vi "Lambda_Configuration_ex_versao1.vi"() -> ()   [LabVIEW 2015]
uses:
  <vilib>/Utility/error.llb/DialogType.ctl
  <vilib>/Utility/file.llb/Read From Spreadsheet File (DBL).vi
  <vilib>/Utility/NIReport.llb/NI_report.lvclass
  <vilib>/addons/_office/NI_ReportGenerationToolkit.lvlib
panel:
  in  "LED Measurement":dbl
  out "error out":errorcluster
  in  "report file path":path=path "C:/Users/Tulio/Documents/Testes/Backup excel/backup excel.xlsx"
  out "Voltage":dbl[](graph)
  out "Current":dbl[](graph)
  in  "Load File?":bool
  in  "?":bool
  out "Output Current":dbl format="%.6f"
  out "Output Voltage":dbl format="%.6f"
  out "Serial Number:":string
  out "error?":bool
  out "Model:":string
  in  "Reset (T)":bool=TRUE
  in  "BAUD":u16(ring)=3 items=["1200", "2400", "4800", "9600", "19200"]
  in  "GEN Addr":i16=6
  in  "VISA name":refnum<visa-resource-name>
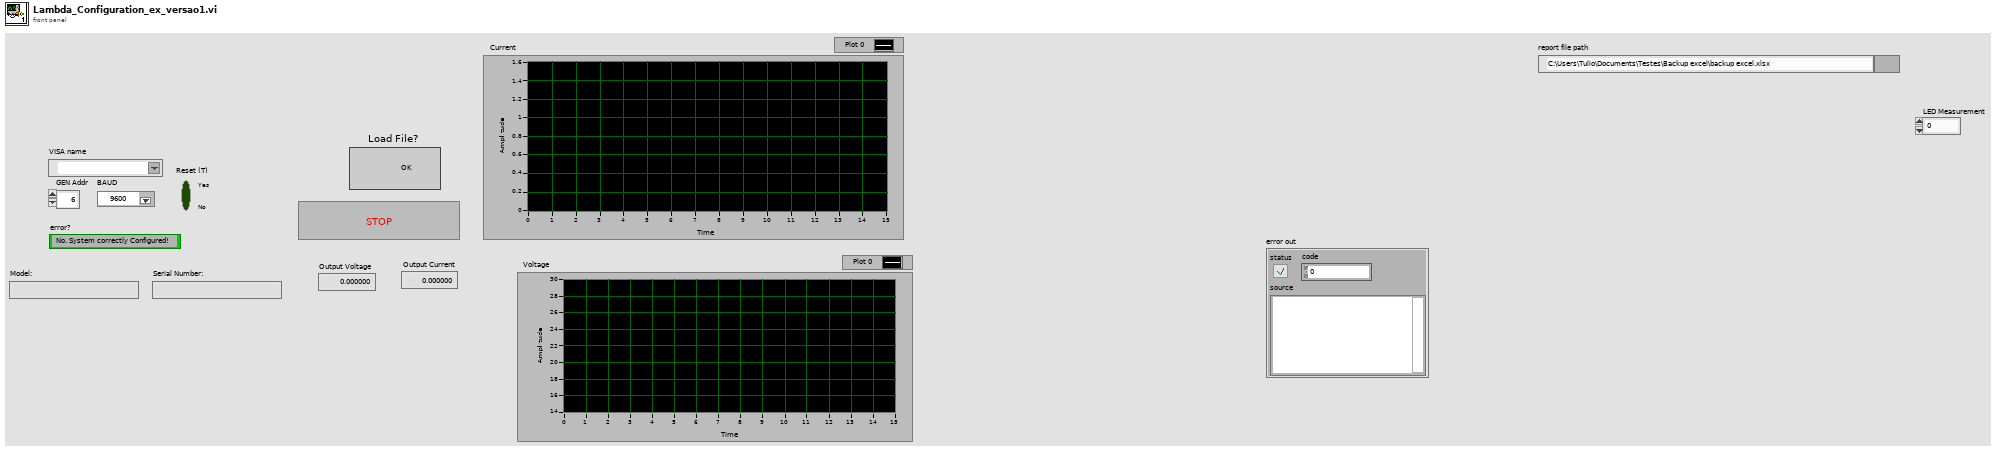
[diagram p1: front panel]
types:
  T1 = enum16{"Standard Report", "HTML", "Word", "Excel"}
  T2 = typedef "DialogType.ctl" = u16
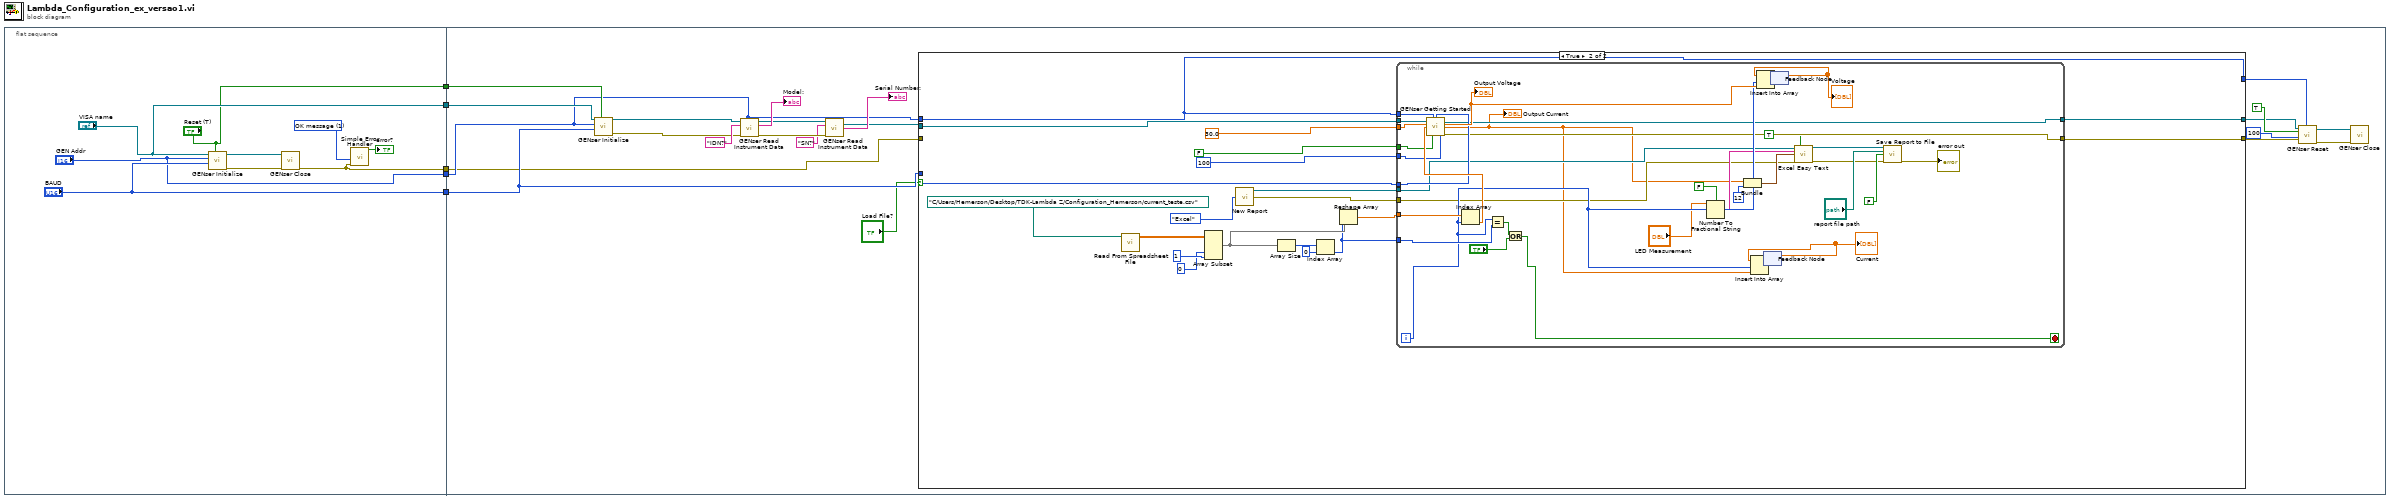
[diagram p0: block diagram]
diagram:
  n1 = flat-sequence {
    tunnel: ["BAUD"] -> w5
    tunnel: ["GEN Addr"] -> w4
    tunnel: ["VISA name"] -> w3
    tunnel: ["Reset (T)"] -> w2
    tunnel: [w6] -> w1
    tunnel: w5 -> [w20]
    tunnel: w4 -> [w22]
    tunnel: w3 -> [w29]
    tunnel: w2 -> [w30]
    tunnel: w1 -> [w15]
    frame #0 {
      w12 = T2 1 items=["no dialog", "OK message", "continue or stop message", "OK message + warnings", "continue/stop + warnings"] ("type of dialog (OK msg:1)")
      n2 = call <instrlib>:"GENser Initialize.vi"("Reset (T)"="Reset (T)", "BAUD"="BAUD", "GEN Addr"="GEN Addr", "VISA name"="VISA name") -> ("error out"=w13:errorcluster, "VISA out"=w14:refnum<visa-resource-name>)  [unwired: 6 in]
      n3 = call <instrlib>:"GENser Close.vi"("error"=w13, "VISA name"=w14) -> ("error out"=w6:errorcluster)  [unwired: 9 in]
      n4 = call <vilib>:"Simple Error Handler.vi"("type of dialog (OK msg:1)"=w12, "error in (no error)"=w6) -> ("error?"=→"error?":bool)  [unwired: 3 in, 4 out]
    }
    frame #1 {
      n5 = call <instrlib>:"GENser Initialize.vi"("Reset (T)"=w30, "BAUD"=w20, "GEN Addr"=w22, "VISA name"=w29) -> ("error out"=w27:errorcluster, "VISA out"=w28:refnum<visa-resource-name>)  [unwired: 6 in]
      n6 = call <instrlib>:"GENser Read Instrument Data.vi"("GEN Addr"=w22, "error"=w27, "Query"="IDN?", "VISA"=w28) -> ("error out"=w33:errorcluster, "Response"=→"Model:":string, "VISA out"=w34:refnum<visa-resource-name>)  [unwired: 4 in, 1 out]
      n7 = call <instrlib>:"GENser Read Instrument Data.vi"("error"=w33, "Query"="SN?", "VISA"=w34) -> ("Response"=→"Serial Number:":string, "VISA out"=w21:refnum<visa-resource-name>)  [unwired: 5 in, 2 out]
      n8 = case shown="True" "Load File?" {
        tunnel: w22 -> [w39 w48]
        tunnel: w21 -> [w38 w49]
        tunnel: w20 -> [_ w52]
        tunnel: [w37 w44] -> w19
        tunnel: [w38 w43] -> w18
        tunnel: [w39 w48] -> w17
        tunnel: w15 -> [w37 _]
        frame False {
        }
        frame True {
          n9 = call-poly <vilib>:"Read From Spreadsheet File.vi"("file path (dialog if empty)"=path "C:/Users/Hemerson/Desktop/TDK-Lambda Z/Configuration_Hemerson/current_teste.csv") -> ("all rows"=w54:dbl[][])  [unwired: 6 in, 4 out]
          n10 = Array Subset "Array Subset"(array=w54, index (col)=0 ("index"), length (col)=1 ("length")) -> (w56:dbl[][])  [unwired: 2 in]
          n11 = call <vilib>:"New Report.vi"("report type"=T1."Excel") -> ("report out"=w41:refnum<class "NI_report.lvclass">, "error out"=w40:errorcluster)  [unwired: 13 in]
          n12 = Array Size(array=w56) -> (size(s)=w57:i32[])
          n13 = Index Array "Index Array"(array=w57, index=0) -> (element=w45:i32)
          n14 = Reshape Array "Reshape Array"(w56, w45) -> (w46:dbl[])
          n15 = while {
            tunnel: w52 -> [w89]
            tunnel: u32 100 ("Settle (0 mS)") -> [w88]
            tunnel: FALSE ("Reset (T)") -> [w87]
            tunnel: w49 -> [w86]
            tunnel: w48 -> [w85]
            tunnel: 30.0 ("Voltage Limit") -> [w84]
            tunnel: w46 -> [w83]
            tunnel: w45 -> [w82]
            tunnel: [w80] -> w44
            tunnel: [w79] -> w43
            tunnel: w41 -> [w66]
            tunnel: w40 -> [w65]
            i -> [w81]
            stop <- w78 stop-if-true
            n16 = Index Array(array=w83, index=w81) -> (element=w90:dbl)
            n17 = call <instrlib>:"GENser Getting Started.vi"("VISA"=w86, "GEN Addr"=w85, "BAUD"=w89, "Voltage Limit"=w84, "Current Limit"=w90, "Reset (T)"=w87, "Settle (0 mS)"=w88) -> ("VISA out"=w79:refnum<visa-resource-name>, "Output Voltage"=w93:dbl, "Output Current"=w64:dbl, "error out"=w80:errorcluster)  [unwired: 5 in]
            "Output Current" <- w64
            "Output Voltage" <- w93
            n18 = Equal?(x=w81, y=w82) -> (x = y?=w91:bool)
            n19 = Or(x=w91, y="?") -> (x .or. y?=w78:bool)
            n20 = Number To Fractional String(use system decimal point (T)=FALSE, number="LED Measurement") -> (F-format string=w67:string)  [unwired: 2 in]
            n21 = Bundle("Output Current"=w64, "offset (0)"=12) -> (w72:cluster{"Output Current":dbl, "offset (0)":i32})  [unwired: 1 in]
            n22 = feedback #1() -> (w62:dbl[])  [unwired: 1 in]
            "Current" <- w62
            n23 = Insert Into Array(array=w62, index=w81, new element=w64) -> (w63:dbl[])
            n24 = feedback-in #1(w63) -> ()
            n25 = feedback #2() -> (w60:dbl[])  [unwired: 1 in]
            "Voltage" <- w60
            n26 = Insert Into Array(array=w60, index=w81, new element=w93) -> (w61:dbl[])
            n27 = feedback-in #2(w61) -> ()
            n28 = call <vilib>:"Excel Easy Text.vi"("report in"=w66, "border? (F)"=TRUE, "text"=w67, "start (-1, -1)"=w72, "error in (no error)"=w65) -> ("report out"=w69:refnum<class "NI_report.lvclass">, "error out"=w70:errorcluster)  [unwired: 6 in, 3 out]
            n29 = call-dynamic "Save Report to File.vi"("report in"=w69, "report file path"="report file path", "prompt to replace? (F)"=FALSE, "error in (no error)"=w70) -> ("error out"=→"error out":errorcluster)  [unwired: 10 in, 1 out]
          }
        }
      }
      n30 = call <instrlib>:"GENser Reset.vi"("GEN Addr"=w17, "error"=w19, "Settle (0 mS)"=u32 100, "Reset (T)"=TRUE, "VISA"=w18) -> ("error out"=w23:errorcluster, "VISA out"=w25:refnum<visa-resource-name>)  [unwired: 5 in]
      n31 = call <instrlib>:"GENser Close.vi"("error"=w23, "VISA name"=w25) -> ()  [unwired: 9 in, 1 out]
    }
  }
